vi "Decode Words to Parameters.vi"(7 "parameters":T1[](array[typedef]), 11 "data words":u16[](array[numeric])=array[4097 elements] format="%04x") -> (3 "Values":dbl[](array[numeric]))   [LabVIEW 2020, in "AIM MIL-STD-1553 Engine.lvlib" / "Implementation.lvlib" / "Rx Execution Unit.lvclass"]
uses:
  Rx Execution Unit.lvclass
  Rx Execution Unit.lvclass/Rx Execution Unit.ctl
  ca490045-0663-4c1d-9dd7-dd62b547f54e.vi
  6fc06d2a-8a23-482f-8d19-e5aba1920577.vi
  Shared/Parameter Definition.ctl
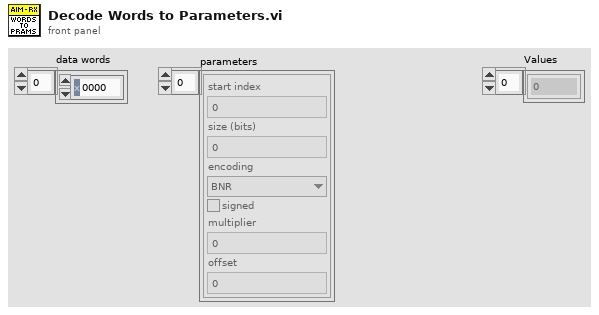
[diagram p1: front panel]
types:
  T1 = typedef "Parameter Definition.ctl" = cluster{"start index":i32, "size (bits)":i32, "encoding":enum16{"BNR", "BCD", "Discrete"}, "signed":bool, "multiplier":dbl, "offset":dbl}
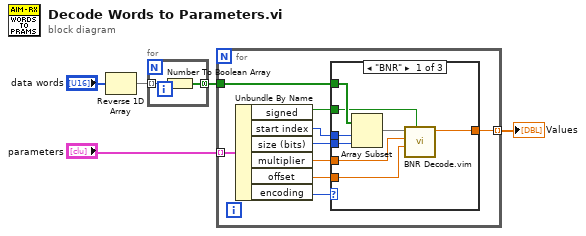
[diagram p0: block diagram]
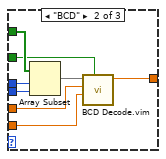
[diagram p2: hidden frame]
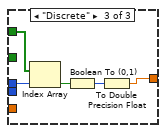
[diagram p3: hidden frame]
diagram:
  n1 = Reverse 1D Array(array="data words") -> (reversed array=w1:u16[])
  n2 = for {
    tunnel: w1 -> [w7] mode=indexing
    tunnel: [w6] -> w3 mode=concatenating
    n3 = Number To Boolean Array(number=w7) -> (Boolean array=w6:bool[])
  }
  n4 = for {
    tunnel: "parameters" -> [w16] mode=indexing
    tunnel: w3 -> [w12]
    tunnel: [w9] -> w4 mode=indexing
    n5 = Unbundle By Name(w16) -> ("signed"=w8:bool, "start index"=w11:i32, "size (bits)"=w10:i32, "multiplier"=w14:dbl, "offset"=w13:dbl, "encoding"=w15:enum16{"BNR", "BCD", "Discrete"})
    n6 = case shown="\"BNR\"" w15 {
      tunnel: w8 -> [w20 w25 _]
      tunnel: w14 -> [w21 w27 _]
      tunnel: w13 -> [w18 w26 _]
      tunnel: w12 -> [w24 w32 w36]
      tunnel: w11 -> [w23 w31 w37]
      tunnel: w10 -> [w22 w30 _]
      tunnel: [w17 w28 w33] -> w9
      frame "BNR" {
        n7 = Array Subset(array=w24, index=w23, length=w22) -> (w19:bool[])
        n8 = call "BNR Decode.vim"("signed"=w20, "scale offset"=w18, "scale multiplier"=w21, "BNR encoded value"=w19) -> ("value"=w17:dbl)  [unwired: 7 in]
      }
      frame "BCD" {
        n9 = Array Subset(array=w32, index=w31, length=w30) -> (w29:bool[])
        n10 = call "BCD Decode.vim"("signed"=w25, "scale offset"=w26, "scale multiplier"=w27, "BCD encoded value"=w29) -> ("value"=w28:dbl)  [unwired: 7 in]
      }
      frame "Discrete" {
        n11 = Index Array(array=w36, index=w37) -> (element=w34:bool)
        n12 = Boolean To (0,1)(Boolean=w34) -> (0, 1=w35:i16)
        n13 = To Double Precision Float(number=w35) -> (double precision float=w33:dbl)
      }
    }
  }
  "Values" <- w4
